vi "Loop_HW.vi"() -> ()   [LabVIEW 2017, in "MechamunDrive.lvlib"]
uses:
  MechamunDrive.lvlib
  Globals/Global_STOP.vi
  Global_SM Out Data.vi
  Global_HW_Status Out.vi
  TypeDefs/Cluster_SRX Status With Encoder.ctl
  Cluster_HW Status.ctl
  Globals/Global_HW_Address_Assignments.vi
  TypeDefs/Cluster_SRX PID Values.ctl
  Enum_HW Cmd Select.ctl
  Cluster_SM to HW Data.ctl
panel:
  in  "HW OVERIDE":bool
  in  "Cmd Display":T1
  in  "Left Right PID Values":T3
  in  "Fwd Back PID Values":T3
  out "Drive Wheel Status":T4
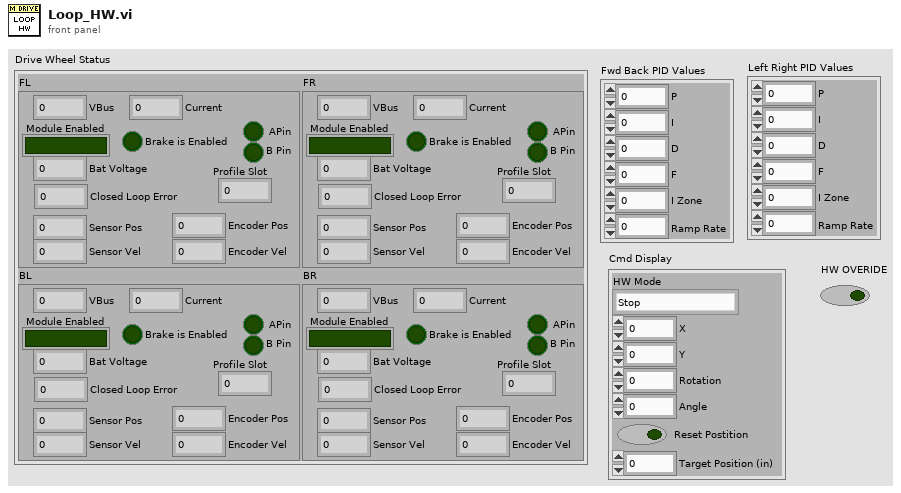
[diagram p1: front panel]
types:
  T1 = typedef "MechamunDrive.lvlib/Cluster_SM to HW Data.ctl" = cluster{"HW Mode":T2, "X":dbl, "Y":dbl, "Rotation":dbl, "Angle":dbl, "Reset Postition":bool, "Target Position (in)":dbl}
  T2 = typedef "MechamunDrive.lvlib/Enum_HW Cmd Select.ctl" = enum16{"Stop", "Vbus", "Positon Lateral", "Postition  FrontBack"}
  T3 = typedef "Cluster_SRX PID Values.ctl" = cluster{"P":dbl, "I":dbl, "D":dbl, "F":dbl, "I Zone":dbl, "Ramp Rate":dbl}
  T4 = typedef "MechamunDrive.lvlib/Cluster_HW Status.ctl" = cluster{"BL":T5, "BR":T5, "FL":T5, "FR":T5}
  T5 = typedef "Cluster_SRX Status With Encoder.ctl" = cluster{"VBus ":dbl, "Module Enabled":bool, "Closed Loop Error":dbl, "Sensor Pos":dbl, "Sensor Vel":dbl, "Current":dbl, "Brake is Enabled":bool, "Encoder Pos":dbl, "Encoder Vel":dbl, " APin":bool, "B Pin":bool, "Bat Voltage":dbl, "Profile Slot":dbl}
  T6 = cluster{"Rear Left Motor ":u8, "Invert Rear Left":bool, "Rear Right Motor":u8, "Invert Rear Right":bool, "Front Left Motor":u8, "Invert Front Left":bool, "Front Right Motor":u8, "Invert Front Right":bool}
  T7 = typedef "WPI_RobotDriveDevRef.ctl" = cluster{"DevStatus":errorcluster, "Motors[]":T8[], "Square Inputs":bool, "Max Output":dbl}
  T8 = typedef "WPI_MotorControlDeviceRef.ctl" = cluster{"DeviceStatus":errorcluster, "Type":T9, "PWM":cluster{"PWM Channel":T10, "DeadBand":T11}, "CAN":cluster{"Device Number":u8, "SetOutput VI Ref":variant, "GetOutput VI Ref":variant, "Enable VI Ref":variant, "Disable VI Ref":variant, "Data":variant}, "Invert":bool, "DIO PWM":cluster{"PWM \"Enable\" Channel":T10, "DIOChannel":T12, "PWM Rate":dbl}}
  T9 = typedef "WPI_MotorControlType.ctl" = enum16{"PWM", "CAN", "DIO PWM"}
  T10 = typedef "FPGA_DIOPWMChannel.ctl" = enum8{"PWM 0", "PWM 1", "PWM 2", "PWM 3", "PWM 4", "PWM 5", "PWM 6", "PWM 7", "PWM 8", "PWM 9", "PWM MXP 0", "PWM MXP 1", "PWM MXP 2", "PWM MXP 3", "PWM MXP 4", "PWM MXP 5", "PWM MXP 6", "PWM MXP 7", "PWM MXP 8", "PWM MXP 9", "Invalid"}
  T11 = typedef "WPI_PWMDeadband.ctl" = cluster{"Name":string, "maxPositivePwm":i32, "minPositivePwm":i32, "centerPwm":i32, "maxNegativePwm":i32, "minNegativePwm":i32, "angularRange":u16}
  T12 = typedef "FPGA_DIOChannel.ctl" = enum8{"DIO 0", "DIO 1", "DIO 2", "DIO 3", "DIO 4", "DIO 5", "DIO 6", "DIO 7", "DIO 8", "DIO 9", "DIO MXP 0", "DIO MXP 1", "DIO MXP 2", "DIO MXP 3", "DIO MXP 4", "DIO MXP 5", "DIO MXP 6", "DIO MXP 7", "DIO MXP 8", "DIO MXP 9", "DIO MXP 10", "DIO MXP 11", "DIO MXP 12", "DIO MXP 13", "DIO MXP 14", "DIO MXP 15", "SPI Port CS1", "SPI Port CS2", "SPI Port CS3", "SPI Port MISO", "SPI Port MOSI", "Invalid"}
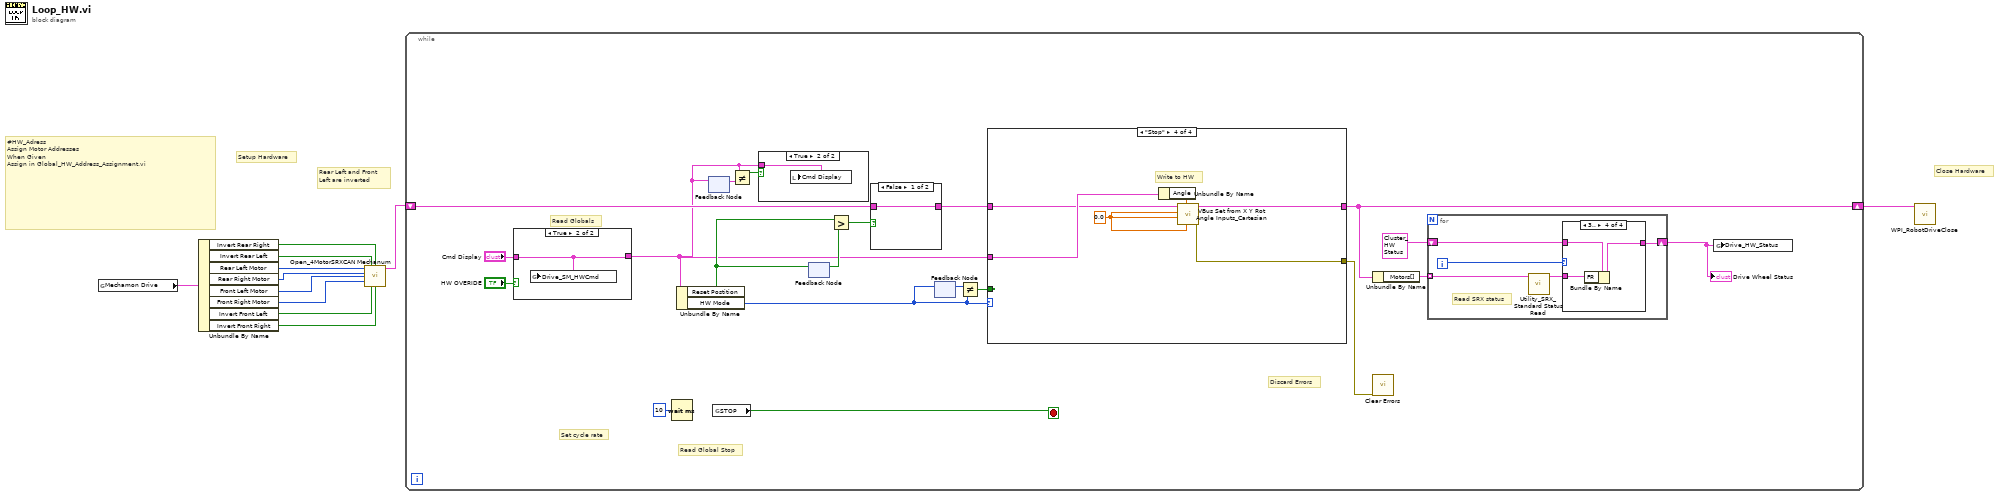
[diagram p0: block diagram]
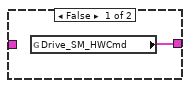
[diagram p2: hidden frame]
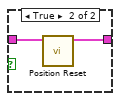
[diagram p4: hidden frame]
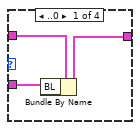
[diagram p5: hidden frame]
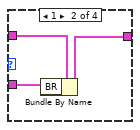
[diagram p6: hidden frame]
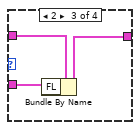
[diagram p7: hidden frame]
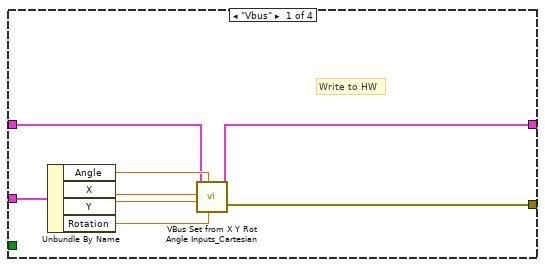
[diagram p8: hidden frame]
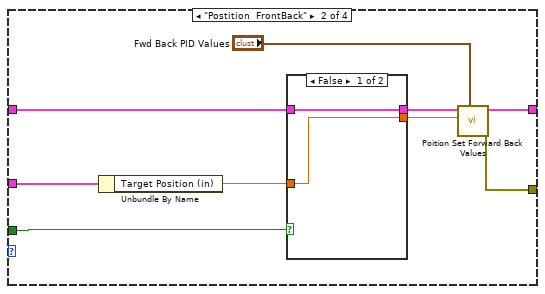
[diagram p9: hidden frame]
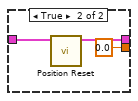
[diagram p10: hidden frame]
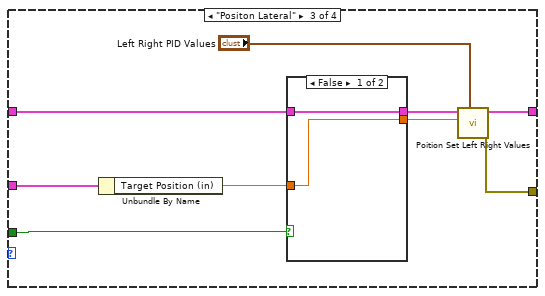
[diagram p11: hidden frame]
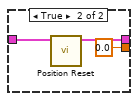
[diagram p12: hidden frame]
diagram:
  # "#HW_Adress\nAssign Motor Addresses\nWhen Given\nAssign in Global_HW_Address_Assignment.vi"
  # "Rear Left and Front \nLeft are inverted"
  # "Close Hardware"
  # "Setup Hardware"
  n1 = global read "Global_HW_Address_Assignments.vi" "Mechamon Drive"() -> (w9:T6)
  n2 = Unbundle By Name(w9) -> ("Invert Rear Right"=w8:bool, "Invert Rear Left"=w7:bool, "Rear Left Motor"=w6:u8, "Rear Right Motor"=w3:u8, "Front Left Motor"=w2:u8, "Front Right Motor"=w1:u8, "Invert Front Left"=w4:bool, "Invert Front Right"=w5:bool)
  n3 = call "Open_4MotorSRXCAN Mechanum.vi"("Rear Left Motor"=w6, "Rear Left Motor Inverted"=w7, "Rear Right Motor Inverted"=w8, "Rear Right Motor"=w3, "Front Left Motor"=w2, "Front Right Motor"=w1, "Front Left Motor Inverted"=w4, "Front Right Motor Inverted"=w5) -> ("RobotDriveDevRef"=w11:T7)  [unwired: 6 in, 1 out]
  n4 = while {
    shift-right: [w27] -> w10
    shift-left: w11 -> [w21]
    stop <- w30 stop-if-true
    # "Discard Errors"
    # "Read Globals"
    # "Read Global Stop"
    # "Set cycle rate"
    n5 = case shown="True" "HW OVERIDE" {
      tunnel: [w32 w33] -> w14
      tunnel: "Cmd Display" -> [_ w33]
      frame False {
        n6 = global read "Global_SM Out Data.vi" "Drive_SM_HWCmd"() -> (w32:T1)
      }
      frame True {
        n7 = global write "Global_SM Out Data.vi" "Drive_SM_HWCmd"(w33) -> ()
      }
    }
    n8 = Wait (ms)(milliseconds to wait=u32 10) -> ()  [unwired: 1 out]
    n9 = Unbundle By Name(w14) -> ("Reset Postition"=w19:bool, "HW Mode"=w24:T2)
    n10 = feedback #1() -> (w16:T1)  [unwired: 1 in]
    n11 = feedback-in #1(w14) -> ()
    n12 = global read "Global_Stop.vi" "STOP"() -> (w30:bool)
    n13 = Not Equal?(x=w14, y=w16) -> (x != y?=w15:bool)
    n14 = case shown="True" w15 {
      tunnel: w14 -> [_ w34]
      frame False {
      }
      frame True {
        n15 = local write "Cmd Display"(w34) -> ()
      }
    }
    n16 = feedback #2() -> (w18:bool)  [unwired: 1 in]
    n17 = feedback-in #2(w19) -> ()
    n18 = Greater?(x=w19, y=w18) -> (0:w17:bool)
    n19 = case shown="False" w17 {
      tunnel: w21 -> [w35 w37]
      tunnel: [w35 w36] -> w20
      frame False {
      }
      frame True {
        n20 = call "Position Reset.vi"("RobotDriveDevRef in"=w37) -> ("RobotDriveDevRef out"=w36:T7)  [unwired: 9 in, 1 out]
      }
    }
    n21 = feedback-in #3(w24) -> ()
    n22 = feedback #3() -> (w23:T2)  [unwired: 1 in]
    n23 = Not Equal?(x=w23, y=w24) -> (x != y?=w22:bool)
    n24 = case shown="\"Stop\"" w24 {
      tunnel: w20 -> [w55 w68 w82 w94]
      tunnel: [w62 w71 w85 w93] -> w27
      tunnel: [w61 w69 w83 w92] -> w29
      tunnel: w14 -> [w60 w70 w84 w96]
      tunnel: w22 -> [_ w66 w80 _]
      frame "Vbus" {
        # "Write to HW"
        n25 = Unbundle By Name(w60) -> ("Angle"=w59:dbl, "X"=w58:dbl, "Y"=w57:dbl, "Rotation"=w56:dbl)
        n26 = call "VBus Set from X Y Rot Angle Inputs_Cartesian.vi"("Rotation"=w56, "Gyro Angle"=w59, "Y"=w57, "X"=w58, "RobotDriveDevRef"=w55) -> ("Error Out"=w61:errorcluster, "RobotDriveDevRef Out"=w62:T7)  [unwired: 5 in]
      }
      frame "Postition  FrontBack" {
        n27 = Unbundle By Name(w70) -> ("Target Position (in)"=w65:dbl)
        n28 = case shown="False" w66 {
          tunnel: w68 -> [w73 w76]
          tunnel: [w73 w75] -> w67
          tunnel: w65 -> [w72 _]
          tunnel: [w72 0.0 ("Target Position (in)")] -> w64
          frame False {
          }
          frame True {
            n29 = call "Position Reset.vi"("RobotDriveDevRef in"=w76) -> ("RobotDriveDevRef out"=w75:T7)  [unwired: 9 in, 1 out]
          }
        }
        n30 = call "Poition Set Forward Back Values.vi"("Position Fwd Back PID Values"="Fwd Back PID Values", "Relative Fwd Back Postion(in)"=w64, "RobotDriveDevRef"=w67) -> ("Error Out"=w69:errorcluster, "RobotDriveDevRef Out"=w71:T7)  [unwired: 7 in]
      }
      frame "Positon Lateral" {
        n31 = Unbundle By Name(w84) -> ("Target Position (in)"=w79:dbl)
        n32 = case shown="False" w80 {
          tunnel: w82 -> [w87 w90]
          tunnel: [w87 w89] -> w81
          tunnel: w79 -> [w86 _]
          tunnel: [w86 0.0 ("Target Position (in)")] -> w78
          frame False {
          }
          frame True {
            n33 = call "Position Reset.vi"("RobotDriveDevRef in"=w90) -> ("RobotDriveDevRef out"=w89:T7)  [unwired: 9 in, 1 out]
          }
        }
        n34 = call "Poition Set Left Right Values.vi"("Left Right PID Values"="Left Right PID Values", "Relative Fwd Back Postion(in)"=w78, "RobotDriveDevRef"=w81) -> ("Error Out"=w83:errorcluster, "RobotDriveDevRef Out"=w85:T7)  [unwired: 7 in]
      }
      frame "Stop" {
        w91 = 0.0 ("Rotation")
        # "Write to HW"
        n35 = Unbundle By Name(w96) -> ("Angle"=w95:dbl)
        n36 = call "VBus Set from X Y Rot Angle Inputs_Cartesian.vi"("Rotation"=w91, "Gyro Angle"=w95, "Y"=w91, "X"=w91, "RobotDriveDevRef"=w94) -> ("Error Out"=w92:errorcluster, "RobotDriveDevRef Out"=w93:T7)  [unwired: 5 in]
      }
    }
    n37 = call <vilib>:"Clear Errors.vi"("error in (no error)"=w29) -> ()  [unwired: 5 in, 2 out]
    n38 = Unbundle By Name(w27) -> ("Motors[]"=w28:T8[])
    n39 = for {
      tunnel: w28 -> [w42] mode=indexing
      shift-right: [w38] -> w25
      shift-left: T4 {"BL"={"VBus "=0.0, "Module Enabled"=FALSE, "Closed Loop Error"=0.0, "Sensor Pos"=0.0, "Sensor Vel"=0.0, "Current"=0.0, "Brake is Enabled"=FALSE, "Encoder Pos"=0.0, "Encoder Vel"=0.0, " APin"=FALSE, "B Pin"=FALSE, "Bat Voltage"=0.0, "Profile Slot"=0.0}, "BR"={"VBus "=0.0, "Module Enabled"=FALSE, "Closed Loop Error"=0.0, "Sensor Pos"=0.0, "Sensor Vel"=0.0, "Current"=0.0, "Brake is Enabled"=FALSE, "Encoder Pos"=0.0, "Encoder Vel"=0.0, " APin"=FALSE, "B Pin"=FALSE, "Bat Voltage"=0.0, "Profile Slot"=0.0}, "FL"={"VBus "=0.0, "Module Enabled"=FALSE, "Closed Loop Error"=0.0, "Sensor Pos"=0.0, "Sensor Vel"=0.0, "Current"=0.0, "Brake is Enabled"=FALSE, "Encoder Pos"=0.0, "Encoder Vel"=0.0, " APin"=FALSE, "B Pin"=FALSE, "Bat Voltage"=0.0, "Profile Slot"=0.0}, "FR"={"VBus "=0.0, "Module Enabled"=FALSE, "Closed Loop Error"=0.0, "Sensor Pos"=0.0, "Sensor Vel"=0.0, "Current"=0.0, "Brake is Enabled"=FALSE, "Encoder Pos"=0.0, "Encoder Vel"=0.0, " APin"=FALSE, "B Pin"=FALSE, "Bat Voltage"=0.0, "Profile Slot"=0.0}} ("Drive Wheel Status") -> [w39]
      i -> [w40]
      # "Read SRX status"
      n40 = call "Utility_SRX_Standard Status Read.vi"("SingleMotorRef"=w42) -> ("SRX With Encoder Out"=w41:T5)  [unwired: 8 in, 2 out]
      n41 = case shown="3.." w40 {
        tunnel: w41 -> [w43 w46 w49 w52]
        tunnel: w39 -> [w45 w48 w51 w54]
        tunnel: [w44 w47 w50 w53] -> w38
        frame ..0 {
          n42 = Bundle By Name(cluster=w45, "BL"=w43) -> (w44:T4)
        }
        frame 1 {
          n43 = Bundle By Name(cluster=w48, "BR"=w46) -> (w47:T4)
        }
        frame 2 {
          n44 = Bundle By Name(cluster=w51, "FL"=w49) -> (w50:T4)
        }
        frame 3.. {
          n45 = Bundle By Name(cluster=w54, "FR"=w52) -> (w53:T4)
        }
      }
    }
    "Drive Wheel Status" <- w25
    n46 = global write "Global_HW_Status Out.vi" "Drive_HW_Status"(w25) -> ()
  }
  n47 = call <vilib>:"WPI_RobotDriveClose.vi"("RobotDriveDevRef"=w10) -> ()  [unwired: 10 in, 1 out]
